vi "triangle_wave_3.vi"() -> ()   [LabVIEW 2017]
panel:
  out "?":bool
  out "F":dbl
  out "T":dbl
  out "R":dbl
  out "T/2":dbl
  out "T'":dbl
  out "F'":dbl
  in  "amp":dbl
  out "T/amp":dbl
  out "Waveform Chart":dbl(graph)
  out "t":dbl
  out "T(s)":dbl
  in  "f(hz)":dbl
  in  "stop":bool
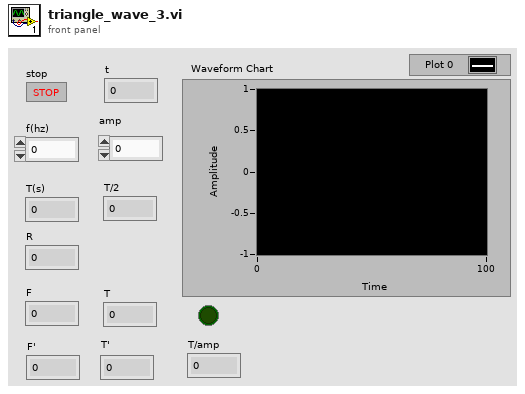
[diagram p1: front panel]
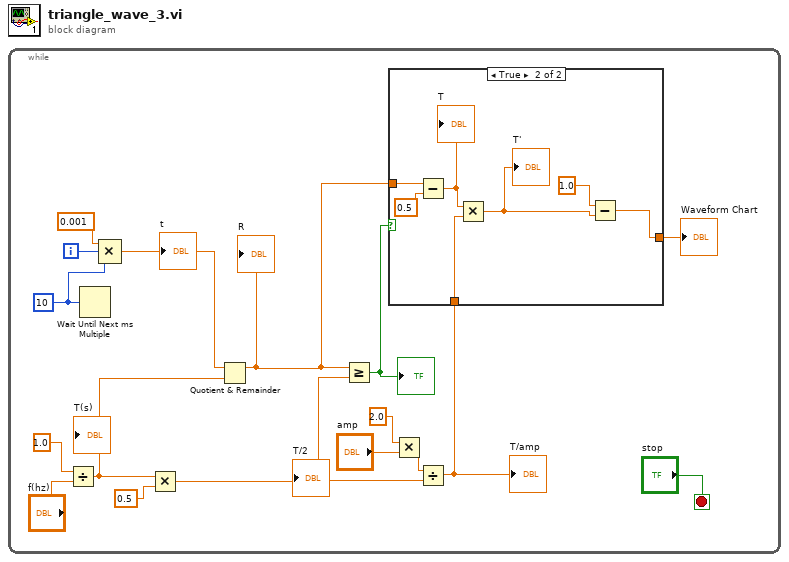
[diagram p0: block diagram]
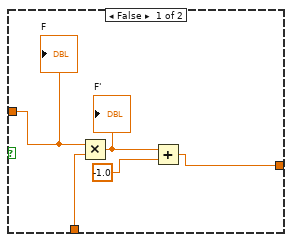
[diagram p2: hidden frame]
diagram:
  n1 = while {
    i -> [w15]
    stop <- "stop" stop-if-true
    w16 = u32 10 ("millisecond multiple")
    n2 = Divide(x=1.0, y="f(hz)") -> (x/y=w2:dbl)
    "T(s)" <- w2
    n3 = Wait Until Next ms Multiple(millisecond multiple=w16) -> ()  [unwired: 1 out]
    n4 = Compound Arithmetic op=MULTIPLY(0.001, w15, w16) -> (w11:dbl)
    "t" <- w11
    n5 = Multiply(x=w2, y=0.5) -> (x*y=w3:dbl)
    "T/2" <- w3
    n6 = Quotient & Remainder(x=w11, y=w2) -> (x-y*floor(x/y)=w1:dbl)  [unwired: 1 out]
    "R" <- w1
    n7 = Greater Or Equal?(x=w1, y=w3) -> (x >= y?=w9:bool)
    "?" <- w9
    n8 = Multiply(x=2.0, y="amp") -> (x*y=w7:dbl)
    n9 = Divide(x=w7, y=w3) -> (x/y=w8:dbl)
    "T/amp" <- w8
    n10 = case shown="True" w9 {
      tunnel: w1 -> [w21 w28]
      tunnel: w8 -> [w22 w29]
      tunnel: [w18 w23] -> w4
      frame False {
        n11 = Multiply(x=w21, y=w22) -> (x*y=w19:dbl)
        "F'" <- w19
        n12 = Add(x=w19, y=-1.0) -> (x+y=w18:dbl)
        "F" <- w21
      }
      frame True {
        n13 = Subtract(x=w28, y=0.5) -> (x-y=w27:dbl)
        "T" <- w27
        n14 = Multiply(x=w27, y=w29) -> (x*y=w24:dbl)
        "T'" <- w24
        n15 = Subtract(x=1.0, y=w24) -> (x-y=w23:dbl)
      }
    }
    "Waveform Chart" <- w4
  }
